vi "Read Digital Display[].vi"(9 "WaveformChart in":refnum<class "WaveformChart.lvclass">) -> (3 "WaveformChart out":refnum<class "WaveformChart.lvclass">, 4 "Digital Display[]":refnum<class "Digital.lvclass">[](array[class]))   [LabVIEW 2014, in "WaveformChart.lvclass"]
uses:
  WaveformChart.lvclass
  Digital/Digital.lvclass
  WaveformChart.lvclass/WaveformChart.ctl
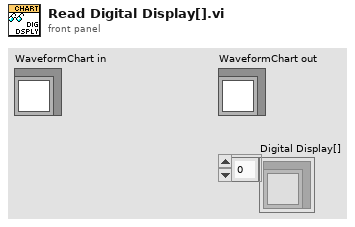
[diagram p1: front panel]
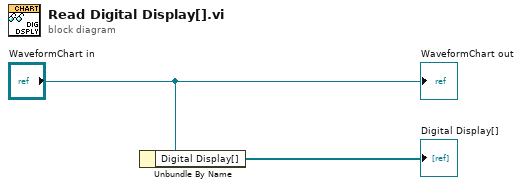
[diagram p0: block diagram]
diagram:
  n1 = Unbundle By Name("WaveformChart in") -> ("Digital Display[]"=→"Digital Display[]":refnum<class "Digital.lvclass">[])
  "WaveformChart out" <- "WaveformChart in"
